vi "MGI Nearest Corners.vi"(2 "Rect 2":T1, 3 "Rect 1":T1) -> (0 "Position 2":cluster{"x":i16, "y":i16}, 1 "Position 1":cluster{"x":i16, "y":i16})   [LabVIEW 2016]
doc: "Find the nearest corners of two rectangles.\n\nAuthored by David A. Moore\nsupport@mooregoodideas.com\nwww.mooregoodideas.com\n\nCopyright (c) 2010, Moore Good Ideas, Inc.\n\nAll rights reserved.\n\nRedistribution and use in source and binary forms, with or without modification, are permitted provided that the following conditions are met:\n\n * Redistributions of source code must retain the above copyright notice, this list of conditions and the following disclaimer.\n * Redistributions in binary form must reproduce the above copyright notice, this list of conditions and the following disclaimer in the documentation and/or other materials provided with the distribution.\n * Neither the name of Moore Good Ideas, Inc. nor the names of its contributors may be used to endorse or promote products derived from this software without specific prior written permission.\n\nTHIS SOFTWARE IS PROVIDED BY THE COPYRIGHT HOLDERS AND CONTRIBUTORS \"AS IS\" AND ANY EXPRESS OR IMPLIED WARRANTIES, INCLUDING, BUT NOT LIMITED TO, THE IMPLIED WARRANTIES OF MERCHANTABILITY AND FITNESS FOR A PARTICULAR PURPOSE ARE DISCLAIMED. IN NO EVENT SHALL THE COPYRIGHT OWNER OR CONTRIBUTORS BE LIABLE FOR ANY DIRECT, INDIRECT, INCIDENTAL, SPECIAL, EXEMPLARY, OR CONSEQUENTIAL DAMAGES (INCLUDING, BUT NOT LIMITED TO, PROCUREMENT OF SUBSTITUTE GOODS OR SERVICES; LOSS OF USE, DATA, OR PROFITS; OR BUSINESS INTERRUPTION) HOWEVER CAUSED AND ON ANY THEORY OF LIABILITY, WHETHER IN CONTRACT, STRICT LIABILITY, OR TORT (INCLUDING NEGLIGENCE OR OTHERWISE) ARISING IN ANY WAY OUT OF THE USE OF THIS SOFTWARE, EVEN IF ADVISED OF THE POSSIBILITY OF SUCH DAMAGE."
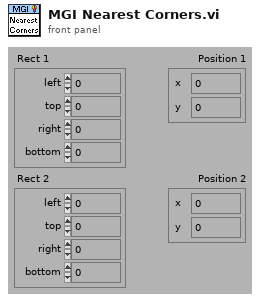
[diagram p1: front panel]
types:
  T1 = cluster{"left":i16, "top":i16, "right":i16, "bottom":i16}
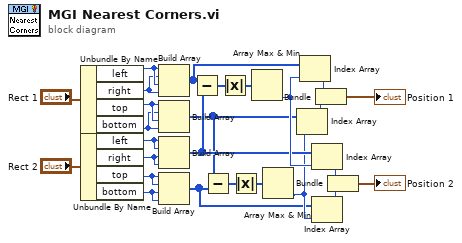
[diagram p0: block diagram]
diagram:
  n1 = Unbundle By Name("Rect 1") -> ("left"=w24:i16, "right"=w23:i16, "top"=w22:i16, "bottom"=w21:i16)
  n2 = Unbundle By Name("Rect 2") -> ("left"=w20:i16, "right"=w19:i16, "top"=w18:i16, "bottom"=w17:i16)
  n3 = Build Array(w24, w23, w24, w23) -> (w12:i16[])
  n4 = Build Array(w22, w21, w22, w21) -> (w9:i16[])
  n5 = Build Array(w20, w20, w19, w19) -> (w10:i16[])
  n6 = Build Array(w18, w18, w17, w17) -> (w7:i16[])
  n7 = Subtract(x=w12, y=w10) -> (x-y=w16:i16[])
  n8 = Subtract(x=w9, y=w7) -> (x-y=w15:i16[])
  n9 = Absolute Value(x=w16) -> (abs(x)=w14:i16[])
  n10 = Absolute Value(x=w15) -> (abs(x)=w13:i16[])
  n11 = Array Max & Min(array=w14) -> (min index (indices)=w11:i32)  [unwired: 3 out]
  n12 = Array Max & Min(array=w13) -> (min index (indices)=w8:i32)  [unwired: 3 out]
  n13 = Index Array(array=w9, index=w8) -> (element=w5:i16)
  n14 = Index Array(array=w12, index=w11) -> (element=w6:i16)
  n15 = Index Array(array=w10, index=w11) -> (element=w3:i16)
  n16 = Index Array(array=w7, index=w8) -> (element=w2:i16)
  n17 = Bundle("right"=w6, "bottom"=w5) -> (→"Position 1":cluster{"right":i16, "bottom":i16})  [unwired: 1 in]
  n18 = Bundle("right"=w3, "bottom"=w2) -> (→"Position 2":cluster{"right":i16, "bottom":i16})  [unwired: 1 in]
